vi "StartPointToEndPoint.vi"() -> (2 "Points":T1[](array[typedef]), 3 "Start Point":T1)   [LabVIEW 2017]
uses:
  KeyPoints.ctl
  DashboardSupport/Startpos.ctl
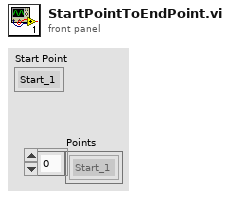
[diagram p1: front panel]
types:
  T1 = typedef "KeyPoints.ctl" = enum16{"Start_1", "Start_2", "Start_3", "Switch_Far", "Switch_Close", "Scale_Far", "Scale_Close", "Cube_1", "Cube_2", "Cube_3", "Cube_4", "Cube_5", "Cube_6", "CubeAcq_Far", "CubeAcq_Close", "Switch_Back_Far", "Switch_Back_Close", "Switch_Side_Far", "Switch_Side_Close"}
  T2 = typedef "Startpos.ctl" = enum16{"Left", "Middle", "Right"}
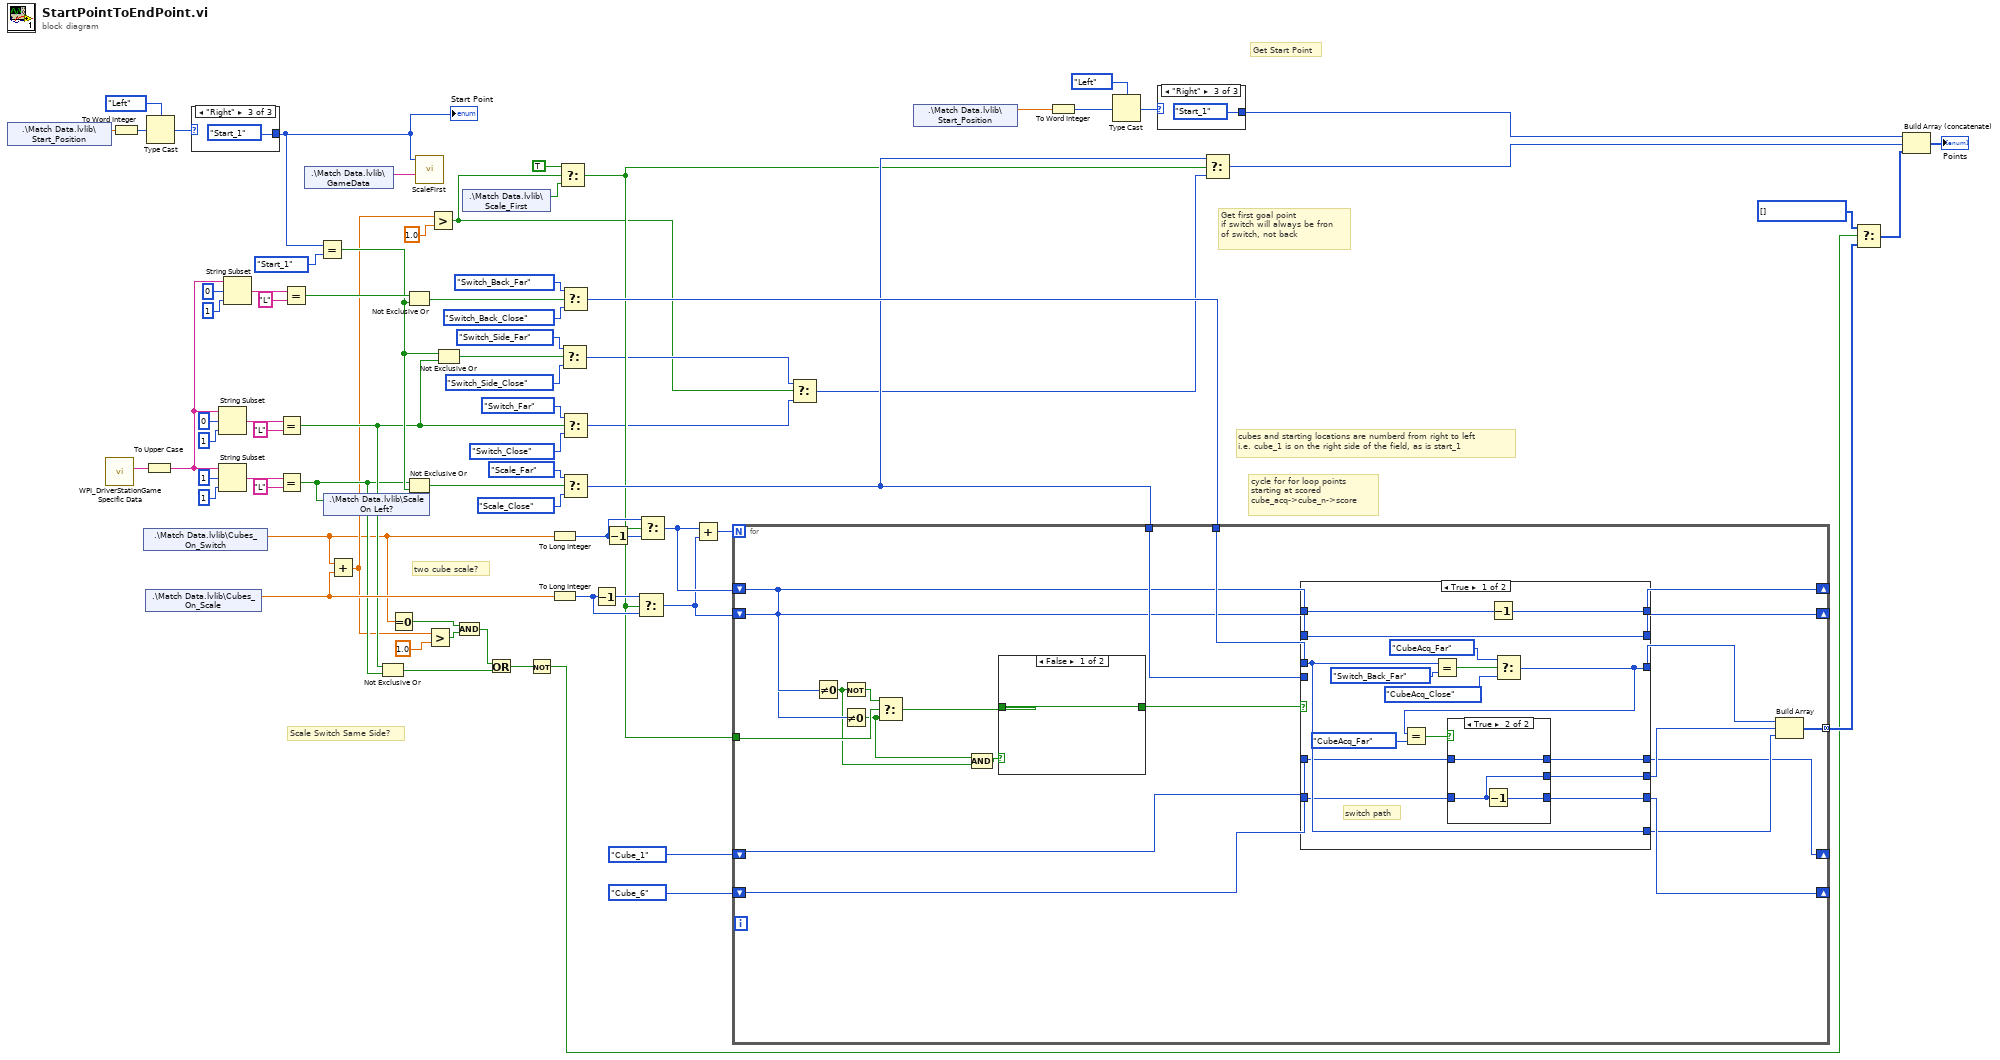
[diagram p0: block diagram]
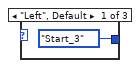
[diagram p2: hidden frame]
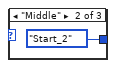
[diagram p3: hidden frame]
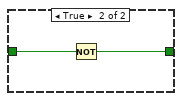
[diagram p4: hidden frame]
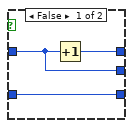
[diagram p5: hidden frame]
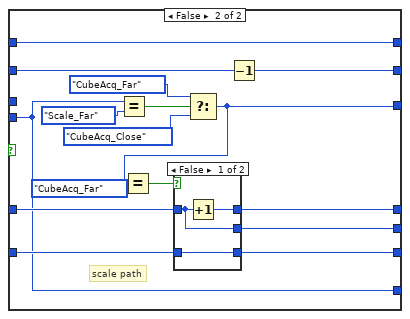
[diagram p6: hidden frame]
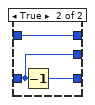
[diagram p7: hidden frame]
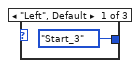
[diagram p8: hidden frame]
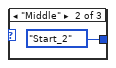
[diagram p9: hidden frame]
diagram:
  w12 = T1[] [] items=["Start_1", "Start_2", "Start_3", "Switch_Far", "Switch_Close", "Scale_Far", "Scale_Close", "Cube_1", "Cube_2", "Cube_3", "Cube_4", "Cube_5", "Cube_6", "CubeAcq_Far", "CubeAcq_Close", "Switch_Back_Far", "Switch_Back_Close", "Switch_Side_Far", "Switch_Side_Close"] ("t")
  # "two cube scale?"
  # "Scale Switch Same Side?"
  # "cubes and starting locations are numberd from right to left\ni.e. cube_1 is on the right side of the field, as is start_1"
  # "cycle for for loop points\nstarting at scored\ncube_acq->cube_n->score"
  # "Get first goal point\nif switch will always be fron\nof switch, not back"
  # "Get Start Point"
  n1 = shared-variable ".\\Match Data.lvlib\\Start_Position"() -> (w33:dbl)  [unwired: 1 in, 1 out]
  n2 = call <vilib>:"WPI_DriverStationGame Specific Data.vi"() -> ("Game Specific Data"=w68:string)  [unwired: 11 in]
  n3 = To Word Integer(number=w33) -> (16bit integer=w34:i16)
  n4 = shared-variable ".\\Match Data.lvlib\\Cubes_On_Switch"() -> (w7:dbl)  [unwired: 1 in, 1 out]
  n5 = To Upper Case(1:w68) -> (0:w51:string)
  n6 = shared-variable ".\\Match Data.lvlib\\Cubes_On_Scale"() -> (w31:dbl)  [unwired: 1 in, 1 out]
  n7 = Type Cast(type=Startpos."Left", x=w34) -> (*(type *) &x=w35:T2)
  n8 = case shown="\"Right\"" w35 {
    tunnel: [KeyPoints."Start_3" ("Start Point") KeyPoints."Start_2" ("Start Point") KeyPoints."Start_1" ("Start Point")] -> w27
    frame "Left", Default {
    }
    frame "Middle" {
    }
    frame "Right" {
    }
  }
  "Start Point" <- w27
  n9 = String Subset(string=w51, offset (0)=0, length (rest)=1 ("length (rest)")) -> (substring=w65:string)
  n10 = String Subset(string=w51, offset (0)=1, length (rest)=1 ("length (rest)")) -> (substring=w62:string)
  n11 = String Subset(string=w51, offset (0)=0, length (rest)=1 ("length (rest)")) -> (substring=w54:string)
  n12 = Equal?(x=w65, y="L") -> (x = y?=w11:bool)
  n13 = Equal?(x=w62, y="L") -> (x = y?=w10:bool)
  n14 = Equal?(x=w54, y="L") -> (x = y?=w25:bool)
  n15 = shared-variable ".\\Match Data.lvlib\\GameData"() -> (w37:string)  [unwired: 1 in, 1 out]
  n16 = Equal?(x=w27, y=KeyPoints."Start_1") -> (x = y?=w16:bool)
  n17 = shared-variable ".\\Match Data.lvlib\\Scale On Left?"(w10) -> ()  [unwired: 1 in, 1 out]
  n18 = Add(x=w7, y=w31) -> (x+y=w9:dbl)
  n19 = Not Exclusive Or(1:w10, 2:w11) -> (0:w3:bool)
  n20 = Equal To 0?(x=w7) -> (x = 0?=w6:bool)
  n21 = Not Exclusive Or(1:w16, 2:w25) -> (0:w24:bool)
  n22 = Not Exclusive Or(1:w16, 2:w10) -> (0:w28:bool)
  n23 = call "ScaleFirst.vi"("Game Data"=w37, "Start Position"=w27) -> ()  [unwired: 9 in, 1 out]
  n24 = Greater?(x=w9, y=1.0) -> (0:w5:bool)
  n25 = Greater?(x=w9, y=1.0 ("x")) -> (0:w18:bool)
  n26 = Not Exclusive Or(1:w11, 2:w16) -> (0:w17:bool)
  n27 = And(x=w6, y=w5) -> (x .and. y?=w4:bool)
  n28 = shared-variable ".\\Match Data.lvlib\\Scale_First"() -> (w29:bool)  [unwired: 1 in, 1 out]
  n29 = Or(x=w4, y=w3) -> (x .or. y?=w2:bool)
  n30 = Not(x=w2) -> (.not. x?=w1:bool)
  n31 = To Long Integer(number=w7) -> (32bit integer=w39:i32)
  n32 = To Long Integer(number=w31) -> (32bit integer=w41:i32)
  n33 = Select(t=TRUE, s=w18, f=w29) -> (s? t:f=w32:bool)
  n34 = Select(t=KeyPoints."Switch_Side_Far" ("Start Point"), s=w17, f=KeyPoints."Switch_Side_Close" ("Start Point")) -> (s? t:f=w21:T1)
  n35 = Select(t=KeyPoints."Switch_Back_Far" ("Start Point"), s=w24, f=KeyPoints."Switch_Back_Close" ("Start Point")) -> (s? t:f=w50:T1)
  n36 = Select(t=KeyPoints."Switch_Far" ("Start Point"), s=w11, f=KeyPoints."Switch_Close" ("Start Point")) -> (s? t:f=w20:T1)
  n37 = Select(t=KeyPoints."Scale_Far" ("Start Point"), s=w28, f=KeyPoints."Scale_Close" ("Start Point")) -> (s? t:f=w49:T1)
  n38 = Decrement(x=w41) -> (x-1=w40:i32)
  n39 = Decrement(x=w39) -> (x-1=w38:i32)
  n40 = Select(t=w40, s=w32, f=w41) -> (s? t:f=w45:i32)
  n41 = Select(t=w39, s=w32, f=w38) -> (s? t:f=w46:i32)
  n42 = Add(x=w46, y=w45) -> (x+y=w47:i32)
  n43 = for {
    N: w47 -> [_]
    tunnel: w49 -> [w98]
    tunnel: w50 -> [w99]
    shift-right: [w96] -> _
    shift-left: w46 -> [w87]
    shift-right: [w97] -> _
    shift-left: w45 -> [w88]
    shift-right: [w94] -> _
    shift-left: KeyPoints."Cube_6" ("Start Point") -> [w95]
    shift-right: [w79] -> _
    shift-left: KeyPoints."Cube_1" ("Start Point") -> [w89]
    tunnel: [w90] -> w14 mode=concatenating
    tunnel: w32 -> [w86]
    n44 = Not Equal To 0?(x=w88) -> (x != 0?=w80:bool)
    n45 = Not(x=w80) -> (.not. x?=w85:bool)
    n46 = Not Equal To 0?(x=w87) -> (x != 0?=w81:bool)
    n47 = Select(t=w85, s=w86, f=w81) -> (s? t:f=w83:bool)
    n48 = Compound Arithmetic op=AND(w81, w80) -> (w82:bool)
    n49 = case shown="False" w82 {
      tunnel: [w100 w102] -> w84
      tunnel: w83 -> [w100 w101]
      frame False {
      }
      frame True {
        n50 = Not(x=w101) -> (.not. x?=w102:bool)
      }
    }
    n51 = case shown="True" w84 {
      tunnel: w87 -> [w118 w140]
      tunnel: w88 -> [w116 w139]
      tunnel: [w116 w125] -> w97
      tunnel: [w117 w140] -> w96
      tunnel: w99 -> [w109 _]
      tunnel: [w111 w134] -> w93
      tunnel: [w109 w126] -> w91
      tunnel: w95 -> [w106 w130]
      tunnel: w89 -> [w107 w131]
      tunnel: [w105 w129] -> w94
      tunnel: [w104 w128] -> w79
      tunnel: [w103 w127] -> w92
      tunnel: w98 -> [_ w126]
      frame True {
        # "switch path"
        n52 = Equal?(x=w109, y=KeyPoints."Switch_Back_Far") -> (x = y?=w114:bool)
        n53 = Decrement(x=w118) -> (x-1=w117:i32)
        n54 = Select(t=KeyPoints."CubeAcq_Far" ("y"), s=w114, f=KeyPoints."CubeAcq_Close" ("y")) -> (s? t:f=w111:T1)
        n55 = Equal?(x=w111, y=KeyPoints."CubeAcq_Far") -> (x = y?=w108:bool)
        n56 = case shown="True" w108 {
          tunnel: w107 -> [w119 w124]
          tunnel: w106 -> [w121 w122]
          tunnel: [w121 w123] -> w105
          tunnel: [w120 w124] -> w104
          tunnel: [w119 w122] -> w103
          frame False {
            n57 = Increment(x=w119) -> (x+1=w120:T1)
          }
          frame True {
            n58 = Decrement(x=w122) -> (x-1=w123:T1)
          }
        }
      }
      frame False {
        # "scale path"
        n59 = Equal?(x=w126, y=KeyPoints."Scale_Far") -> (x = y?=w137:bool)
        n60 = Select(t=KeyPoints."CubeAcq_Far" ("y"), s=w137, f=KeyPoints."CubeAcq_Close" ("y")) -> (s? t:f=w134:T1)
        n61 = Equal?(x=w134, y=KeyPoints."CubeAcq_Far") -> (x = y?=w132:bool)
        n62 = case shown="False" w132 {
          tunnel: w131 -> [w141 w146]
          tunnel: w130 -> [w143 w144]
          tunnel: [w143 w145] -> w129
          tunnel: [w142 w146] -> w128
          tunnel: [w141 w144] -> w127
          frame False {
            n63 = Increment(x=w141) -> (x+1=w142:T1)
          }
          frame True {
            n64 = Decrement(x=w144) -> (x-1=w145:T1)
          }
        }
        n65 = Decrement(x=w139) -> (x-1=w125:i32)
      }
    }
    n66 = Build Array(w93, w92, w91) -> (w90:T1[])
  }
  n67 = Select(t=w21, s=w18, f=w20) -> (s? t:f=w19:T1)
  n68 = shared-variable ".\\Match Data.lvlib\\Start_Position"() -> (w74:dbl)  [unwired: 1 in, 1 out]
  n69 = To Word Integer(number=w74) -> (16bit integer=w42:i16)
  n70 = Type Cast(type=Startpos."Left", x=w42) -> (*(type *) &x=w73:T2)
  n71 = case shown="\"Right\"" w73 {
    tunnel: [KeyPoints."Start_3" ("Start Point") KeyPoints."Start_2" ("Start Point") KeyPoints."Start_1" ("Start Point")] -> w72
    frame "Left", Default {
    }
    frame "Middle" {
    }
    frame "Right" {
    }
  }
  n72 = Select(t=w49, s=w32, f=w19) -> (s? t:f=w48:T1)
  n73 = Select(t=w12, s=w1, f=w14) -> (s? t:f=w13:T1[])
  n74 = Build Array (concatenate)(w72, w48, w13) -> (→"Points":T1[])
